vi "test remove array.vi"() -> ()   [LabVIEW 2017]
uses:
  e32d0ae5-4b0f-4f24-85be-3e077702e35c.vi
panel:
  out "array w/ subset deleted":string[](array[string])
  out "deleted elements":string[](array[string])
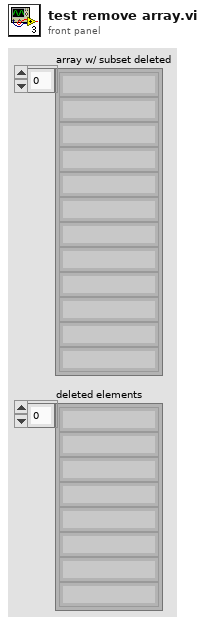
[diagram p1: front panel]
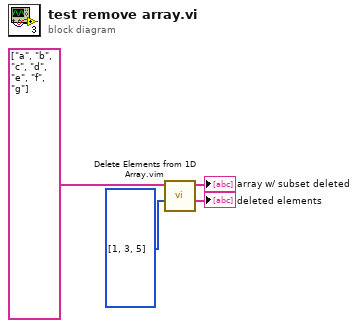
[diagram p0: block diagram]
diagram:
  n1 = call "Delete Elements from 1D Array.vim"("indices"=i32[] [1, 3, 5], "array"=string[] ["a", "b", "c", "d", "e", "f", "g"]) -> ("deleted elements"=→"deleted elements":string[], "array w/ subset deleted"=→"array w/ subset deleted":string[])  [unwired: 8 in]
